vi "Create.vi"(8 "error in (no error)":errorcluster, 10 "plugin configuration":T1={"core"={"name"="", "components"=[], "cycle timing"={"priority"=10000, "decimation"=1, "offset"=0}}, "component settings"=[], "threads"=[]}, 11 "Plugin Configuration in":refnum<class "Plugin Configuration.lvclass">) -> (0 "error out":errorcluster, 3 "Plugin Configuration out":refnum<class "Plugin Configuration.lvclass">)   [LabVIEW 2017, in "DSF Core.lvlib" / "Plugin Configuration.lvclass"]
uses:
  Plugin Configuration.lvclass
  C:/Git/DSF/Core/Classes/Configuration/Runtime/Runtime Configuration.lvclass
  Typedefs/DSF Engine Plugin Configuration.ctl
  Typedefs/DSF Core Plugin Configuration.ctl
  Typedefs/DSF Timing Info.ctl
  Typedefs/DSF Settings Info.ctl
  Typedefs/DSF Version Info.ctl
  Typedefs/DSF Engine Plugin Thread Configuration.ctl
  Typedefs/DSF Core Thread Configuration.ctl
  Typedefs/DSF Engine Transfer Group Configuration.ctl
  Typedefs/DSF Core Group Configuration.ctl
  Typedefs/DSF Direction.ctl
  Typedefs/DSF Timeout Behavior.ctl
  Typedefs/DSF Engine Transfer Configuration.ctl
  Typedefs/DSF Core Transfer Configuration.ctl
  Typedefs/DSF Engine Channel Configuration.ctl
  Typedefs/DSF Core Channel Configuration.ctl
  Typedefs/DSF Data Type.ctl
  Plugin Configuration.lvclass/Plugin Configuration.ctl
  Thread/Thread Configuration.lvclass
  Runtime/Runtime Configuration.lvclass
  DSF Core.lvlib
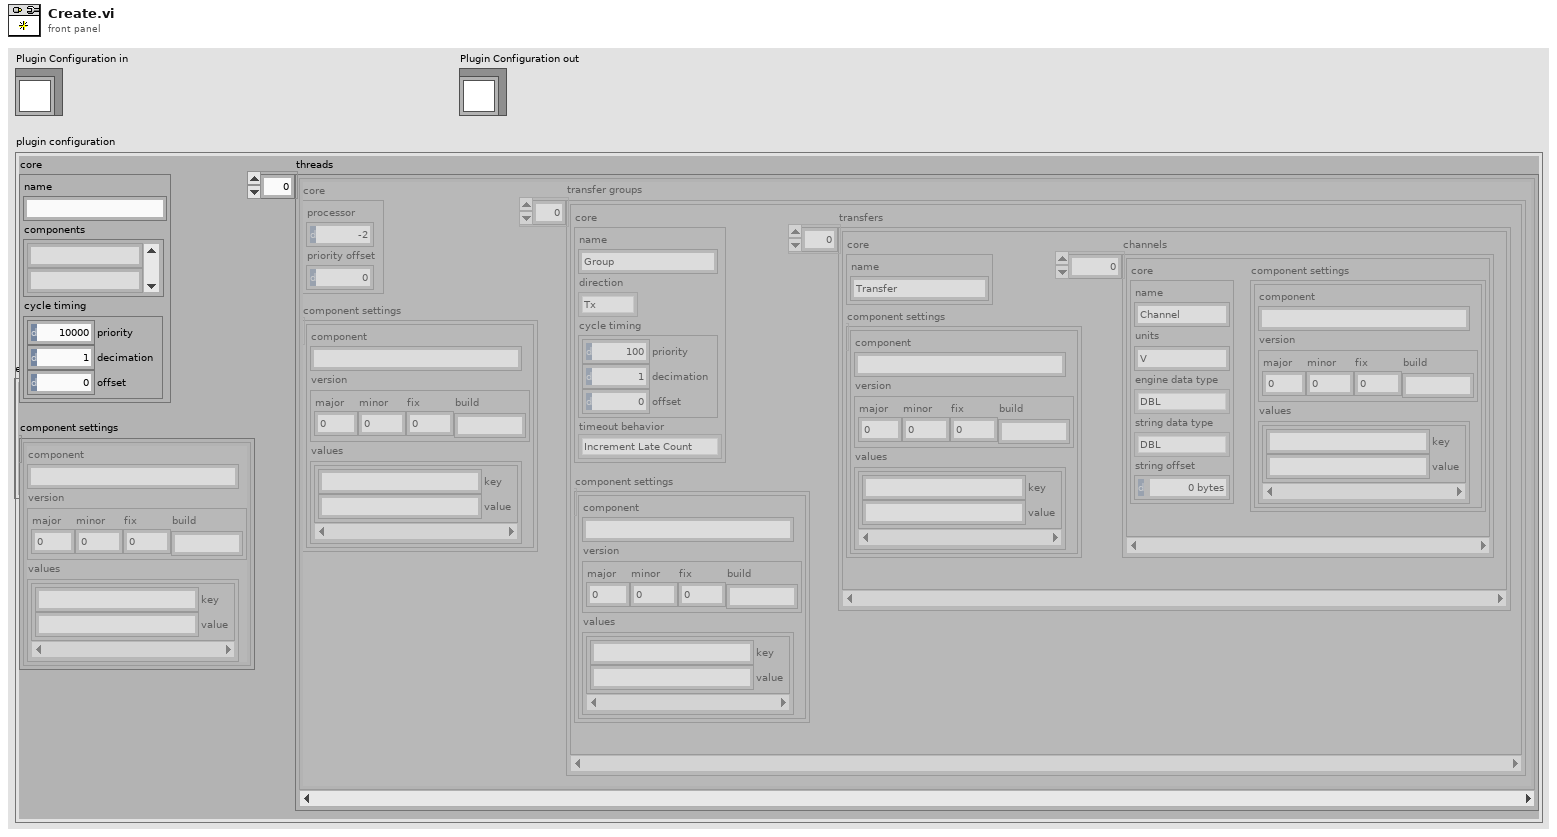
[diagram p1: front panel]
types:
  T1 = typedef "DSF Core.lvlib/DSF Engine Plugin Configuration.ctl" = cluster{"core":T2, "component settings":T4[], "threads":T6[]}
  T2 = typedef "DSF Core.lvlib/DSF Core Plugin Configuration.ctl" = cluster{"name":string, "components":string[], "cycle timing":T3}
  T3 = typedef "DSF Core.lvlib/DSF Timing Info.ctl" = cluster{"priority":u64, "decimation":u64, "offset":u64}
  T4 = typedef "DSF Core.lvlib/DSF Settings Info.ctl" = cluster{"component":string, "version":T5, "values":cluster{"key":string, "value":string}[]}
  T5 = typedef "DSF Core.lvlib/DSF Version Info.ctl" = cluster{"major":u32, "minor":u32, "fix":u32, "build":string}
  T6 = typedef "DSF Core.lvlib/DSF Engine Plugin Thread Configuration.ctl" = cluster{"core":T7, "component settings":T4[], "transfer groups":T8[]}
  T7 = typedef "DSF Core.lvlib/DSF Core Thread Configuration.ctl" = cluster{"processor":i32, "priority offset":i16}
  T8 = typedef "DSF Core.lvlib/DSF Engine Transfer Group Configuration.ctl" = cluster{"core":T9, "component settings":T4[], "transfers":T12[]}
  T9 = typedef "DSF Core.lvlib/DSF Core Group Configuration.ctl" = cluster{"name":string, "direction":T10, "cycle timing":T3, "timeout behavior":T11}
  T10 = typedef "DSF Core.lvlib/DSF Direction.ctl" = enum8{"Tx", "Rx"}
  T11 = typedef "DSF Core.lvlib/DSF Timeout Behavior.ctl" = enum8{"Increment Late Count", "Throw Error"}
  T12 = typedef "DSF Core.lvlib/DSF Engine Transfer Configuration.ctl" = cluster{"core":T13, "component settings":T4[], "channels":T14[]}
  T13 = typedef "DSF Core.lvlib/DSF Core Transfer Configuration.ctl" = cluster{"name":string}
  T14 = typedef "DSF Core.lvlib/DSF Engine Channel Configuration.ctl" = cluster{"core":T15, "component settings":T4[]}
  T15 = typedef "DSF Core.lvlib/DSF Core Channel Configuration.ctl" = cluster{"name":string, "units":string, "engine data type":T16, "string data type":T16, "string offset":u64}
  T16 = typedef "DSF Core.lvlib/DSF Data Type.ctl" = enum8{"Bool", "SGL", "DBL", "I8", "I16", "I32", "I64", "U8", "U16", "U32", "U64"}
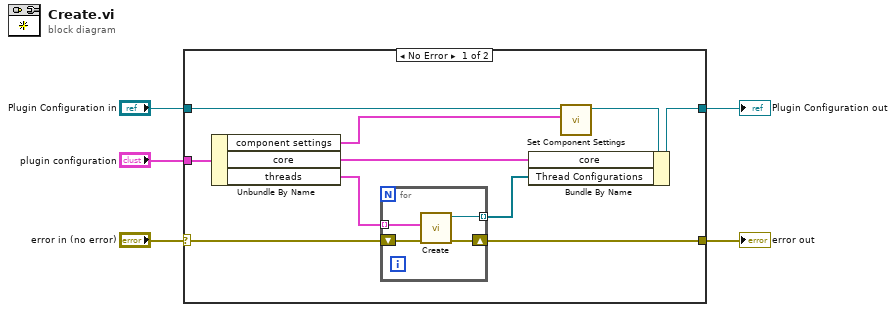
[diagram p0: block diagram]
diagram:
  n1 = case shown="No Error" "error in (no error)" {
    selector: "error in (no error)" -> [w12 w21]
    tunnel: [w11 w21] -> w4
    tunnel: [w15 w20] -> w2
    tunnel: "Plugin Configuration in" -> [w8 w20]
    tunnel: "plugin configuration" -> [w14 _]
    frame No Error {
      n2 = Unbundle By Name(w14) -> ("component settings"=w6:T4[], "core"=w13:T2, "threads"=w10:T6[])
      n3 = for {
        shift-right: [w18] -> w11
        shift-left: w12 -> [w19]
        tunnel: w10 -> [w17] mode=indexing
        tunnel: [w16] -> w9 mode=indexing
        n4 = call "Create.vi"("error in (no error)"=w19, "thread configuration"=w17) -> ("error out"=w18:errorcluster, "Thread Configuration out"=w16:refnum<class "Thread Configuration.lvclass">)  [unwired: 8 in]
      }
      n5 = call "Set Component Settings.vi"("component settings"=w6, "Runtime Configuration in"=w8) -> ("Runtime Configuration out"=w7:refnum<class "Plugin Configuration.lvclass">)  [unwired: 8 in, 1 out]
      n6 = Bundle By Name(cluster=w7, "core"=w13, "Thread Configurations"=w9) -> (w15:refnum<class "Plugin Configuration.lvclass">)
    }
    frame Error {
    }
  }
  "error out" <- w4
  "Plugin Configuration out" <- w2
